vi "CTRE_Phoenix_Pigeon2_GetStickyFaults.vi"(8 "error in":errorcluster, 11 "Pigeon2DevRef 2":T2={"DeviceStatus"={"status"=FALSE, "code"=0, "source"=""}, "Device Number"=0, "Type"=352321536, "Device ID"=0, "Handle"=0, "UsageFrame"=0, "Library Path"=path ""} {"Type" items=["CAN"=352321536, "TalonSRX"=33554432]}) -> (0 "error out":errorcluster, 2 "Faults":T1, 3 "Pigeon2DevRef":T2={"DeviceStatus"={"status"=FALSE, "code"=0, "source"=""}, "Device Number"=0, "Type"=352321536, "Device ID"=0, "Handle"=0, "UsageFrame"=0, "Library Path"=path ""} {"Type" items=["CAN"=352321536, "TalonSRX"=33554432]})   [LabVIEW 2020]
doc: "Gets the Sticky Faults from a Pigeon2."
uses:
  <vilib>/Rock Robotics/WPI/ThirdParty/Phoenix-LabVIEW/Pigeon IMU/CTRE_PigeonIMU_DeviceRef.ctl
  <vilib>/Rock Robotics/WPI/ThirdParty/Phoenix-LabVIEW/Pigeon IMU/CTRE_PigeonIMU_ConnectionType.ctl
  <vilib>/Rock Robotics/WPI/ThirdParty/Phoenix-LabVIEW/Pigeon2/controls/CTRE_Phoenix_Pigeon2_Faults.ctl
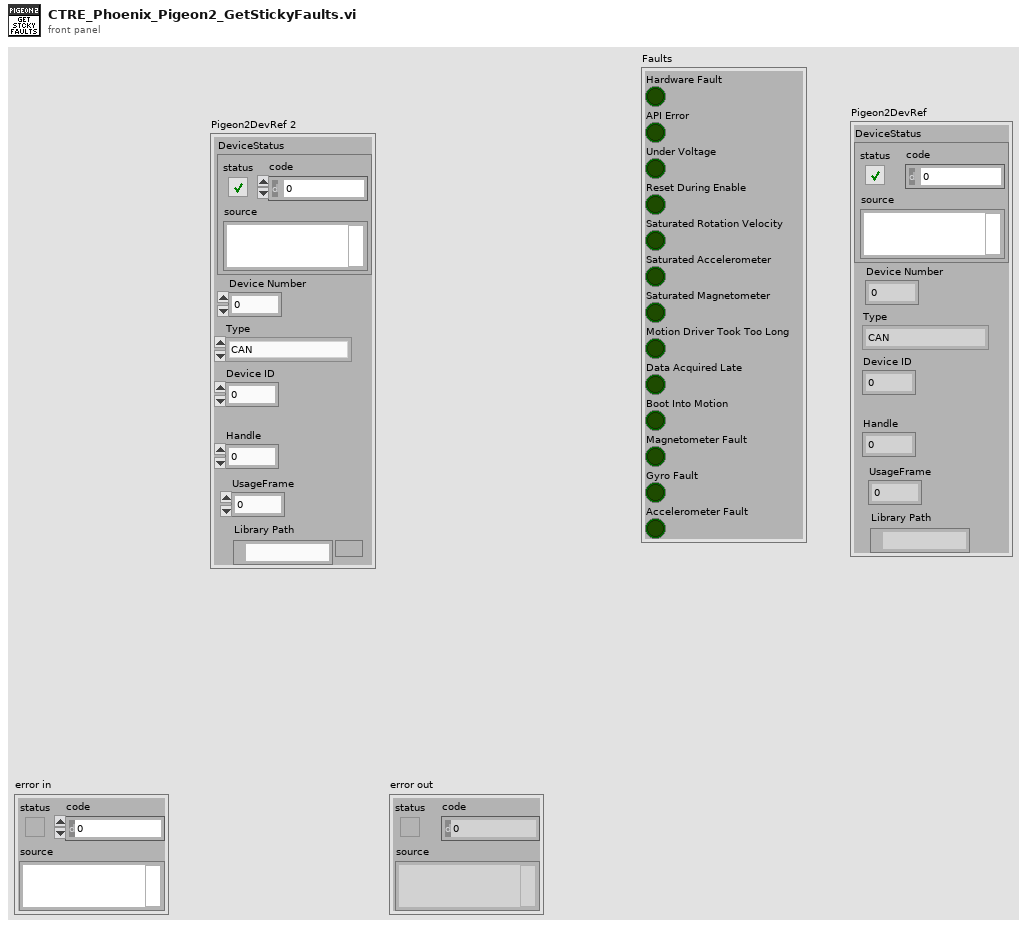
[diagram p1: front panel]
types:
  T1 = typedef "CTRE_Phoenix_Pigeon2_Faults.ctl" = cluster{"Hardware Fault":bool, "API Error":bool, "Under Voltage":bool, "Reset During Enable":bool, "Saturated Rotation Velocity":bool, "Saturated Accelerometer":bool, "Saturated Magnetometer":bool, "Motion Driver Took Too Long":bool, "Data Acquired Late":bool, "Boot Into Motion":bool, "Magnetometer Fault":bool, "Gyro Fault":bool, "Accelerometer Fault":bool}
  T2 = typedef "CTRE_PigeonIMU_DeviceRef.ctl" = cluster{"DeviceStatus":errorcluster, "Device Number":u8, "Type":T3, "Device ID":u32, "Handle":u64, "UsageFrame":u32, "Library Path":path}
  T3 = typedef "CTRE_PigeonIMU_ConnectionType.ctl" = u32
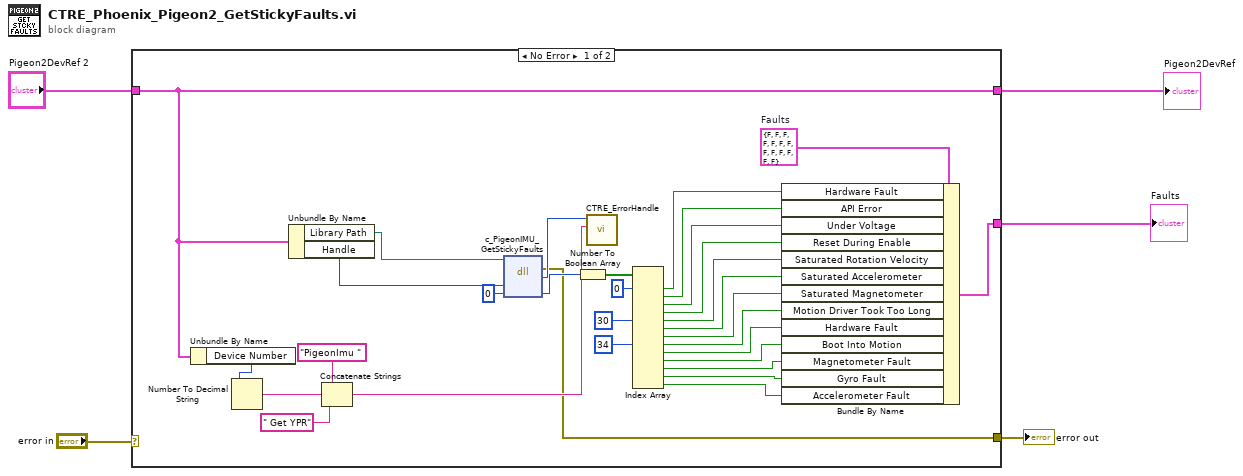
[diagram p0: block diagram]
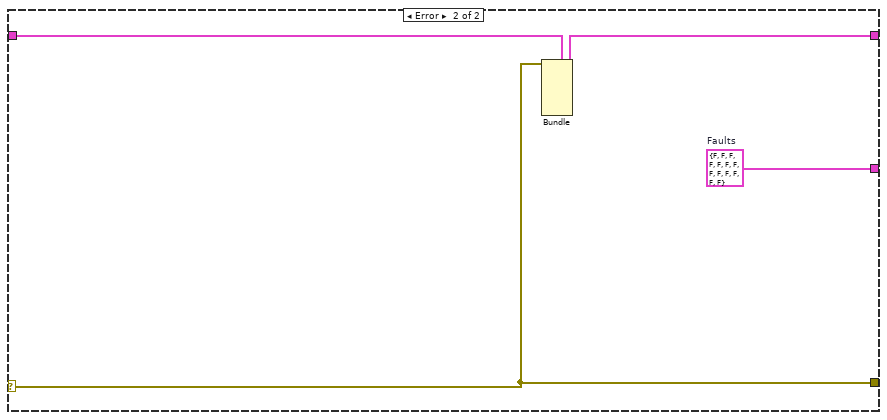
[diagram p2: hidden frame]
diagram:
  n1 = case shown="No Error" "error in" {
    selector: "error in" -> [_ w39]
    tunnel: "Pigeon2DevRef 2" -> [w30 w40]
    tunnel: [w7 w39] -> w5
    tunnel: [w30 w38] -> w2
    tunnel: [w8 w37] -> w1
    frame No Error {
      w24 = T1 {"Hardware Fault"=FALSE, "API Error"=FALSE, "Under Voltage"=FALSE, "Reset During Enable"=FALSE, "Saturated Rotation Velocity"=FALSE, "Saturated Accelerometer"=FALSE, "Saturated Magnetometer"=FALSE, "Motion Driver Took Too Long"=FALSE, "Data Acquired Late"=FALSE, "Boot Into Motion"=FALSE, "Magnetometer Fault"=FALSE, "Gyro Fault"=FALSE, "Accelerometer Fault"=FALSE}  # Faults
      n2 = Unbundle By Name(w30) -> ("Device Number"=w33:u8)
      n3 = Number To Decimal String(number=w33) -> (decimal integer string=w34:string)  [unwired: 1 in]
      n4 = Unbundle By Name(w30) -> ("Library Path"=w29:path, "Handle"=w28:u64)
      n5 = Concatenate Strings("PigeonImu " ("string"), w34, " Get YPR" ("string")) -> (w35:string)
      n6 = dll-call lib="?" fn="c_PigeonIMU_GetStickyFaults"(path in=w29, "handle"=w28, "param"=0) -> (error out=w7:errorcluster, "return type"=w36:i32, "param"=w26:u64)  [unwired: 3 in, 1 out]
      n7 = Number To Boolean Array(number=w26) -> (Boolean array=w25:bool[])
      n8 = call <vilib>:"CTRE_ErrorHandle.vi"("origin"=w35, "code"=w36) -> ()  [unwired: 9 in, 1 out]
      n9 = Index Array(array=w25, index #1=0 ("index"), index #5=30 ("index"), index #8=34 ("index")) -> (element #1=w23:bool, element #2=w22:bool, element #3=w21:bool, element #4=w20:bool, element #5=w17:bool, element #6=w16:bool, element #7=w15:bool, element #8=w14:bool, element #9=w13:bool, element #10=w12:bool, element #11=w11:bool, element #12=w10:bool, element #13=w9:bool)  [unwired: 10 in]
      n10 = Bundle By Name(cluster=w24, "Hardware Fault"=w23, "API Error"=w22, "Under Voltage"=w21, "Reset During Enable"=w20, "Saturated Rotation Velocity"=w17, "Saturated Accelerometer"=w16, "Saturated Magnetometer"=w15, "Motion Driver Took Too Long"=w14, "Hardware Fault"=w13, "Boot Into Motion"=w12, "Magnetometer Fault"=w11, "Gyro Fault"=w10, "Accelerometer Fault"=w9) -> (w8:T1)
    }
    frame Error {
      w37 = T1 {"Hardware Fault"=FALSE, "API Error"=FALSE, "Under Voltage"=FALSE, "Reset During Enable"=FALSE, "Saturated Rotation Velocity"=FALSE, "Saturated Accelerometer"=FALSE, "Saturated Magnetometer"=FALSE, "Motion Driver Took Too Long"=FALSE, "Data Acquired Late"=FALSE, "Boot Into Motion"=FALSE, "Magnetometer Fault"=FALSE, "Gyro Fault"=FALSE, "Accelerometer Fault"=FALSE}  # Faults
      n11 = Bundle(cluster=w40, "DeviceStatus"=w39) -> (w38:T2)  [unwired: 6 in]
    }
  }
  "error out" <- w5
  "Pigeon2DevRef" <- w2
  "Faults" <- w1
